vi "Camera_Crop_X_Axis.vi"(9 "Detect Movement":bool, 10 "Camera":T1, 11 "input cluster":T2 {"SystemVersion" items=["Standard", "XL"]; "Overlay_Ring" items=["Session Data", "Extended Setup", "Buffer", "Camera", "Dispenser", "Stats", "Connections"]; "Flush Size" min=1; "Dispense Speed" min=1; "Rectangle 2"."Rotation" format="%.2f"; "Rectangle 2"."Left" scale=0.0..1024.0; "Rectangle 2"."Right" scale=0.0..1024.0; "Rectangle 1"."Rotation" format="%.2f"; "Rectangle 1"."Left" scale=0.0..1024.0; "Rectangle 1"."Right" scale=0.0..1024.0; "Max Framerate" min=1; "Overload threshold" min=1; "Image Save Queue Size" min=1; "Image Process Queue Size" min=1; "Empty start" min=1; "Sample size threshold" min=1; "Framerate" min=1; "Light intensity" scale=0.0..100.0}) -> (1 "Width":i64, 3 "OffsetX":i64)   [LabVIEW 2021]
uses:
  controls/Data.ctl
  <vilib>/userDefined/High Color/IMAQdx.ctl
  <vilib>/vision/Image Controls.llb/IMAQ Image.ctl
  Camera_ID.ctl
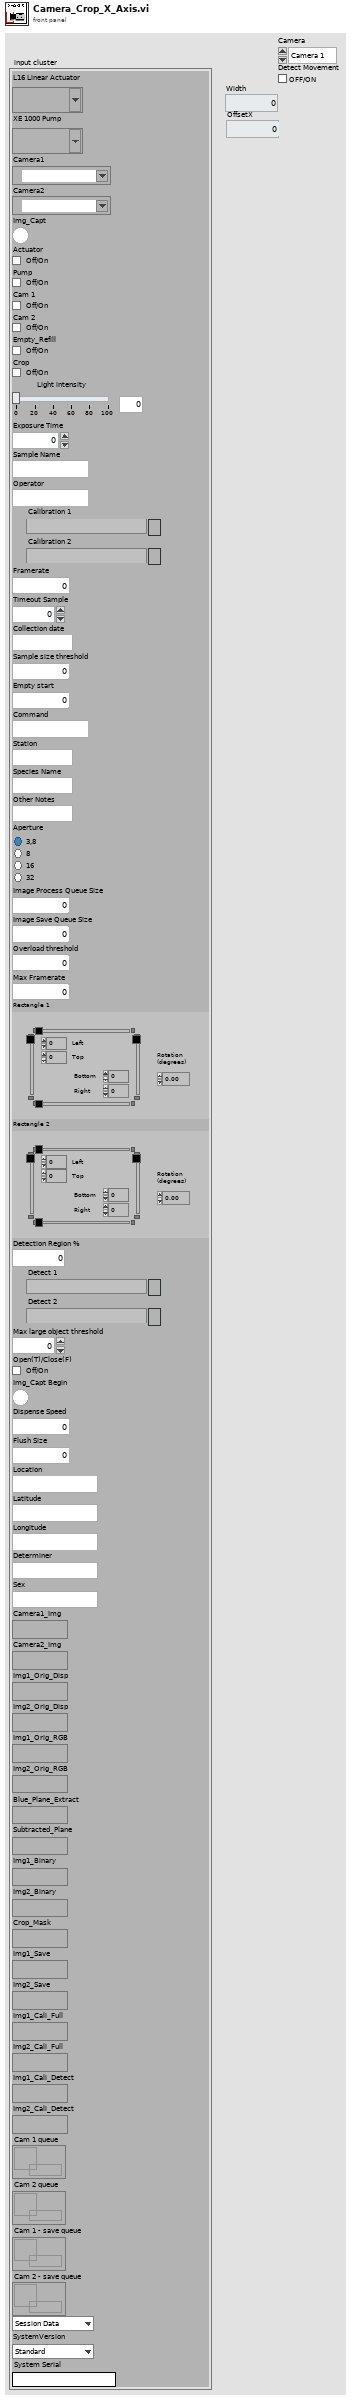
[diagram p1: front panel]
types:
  T1 = typedef "Camera_ID.ctl" = enum16{"Camera 1", "Camera 2"}
  T2 = typedef "Data.ctl" = cluster{"L16 Linear Actuator":refnum<visa-resource-name>, "XE 1000 Pump":refnum<visa-resource-name>, "Camera1":T3, "Camera2":T3, "Img_Capt":bool, "Actuator":bool, "Pump":bool, "Cam 1":bool, "Cam 2":bool, "Empty_Refill":bool, "Crop":bool, "Light intensity":i32, "Exposure Time":dbl, "Sample Name":string, "Operator":string, "Calibration 1":path, "Calibration 2":path, "Framerate":i32, "Timeout Sample":i32, "Collection date":string, "Sample size threshold":i32, "Empty start":u32, "Command":string, "Station":string, "Species Name":string, "Other Notes":string, "Aperture":enum32{"Item 0", "Item 1", "Item 2", "Item 3"}, "Image Process Queue Size":i32, "Image Save Queue Size":i32, "Overload threshold":i32, "Max Framerate":i32, "Rectangle 1":T4, "Rectangle 2":T4, "Detection Region %":dbl, "Detect 1":path, "Detect 2":path, "Max large object threshold":i32, "Open(T)/Close(F)":bool, "Img_Capt Begin":bool, "Dispense Speed":i32, "Flush Size":i32, "Location":string, "Latitude":string, "Longitude":string, "Determiner":string, "Sex":string, "Camera1_Img":T5, "Camera2_Img":T5, "Img1_Orig_Disp":T5, "Img2_Orig_Disp":T5, "Img1_Orig_RGB":T5, "Img2_Orig_RGB":T5, "Blue_Plane_Extract":T5, "Subtracted_Plane":T5, "Img1_Binary":T5, "Img2_Binary":T5, "Crop_Mask":T5, "Img1_Save":T5, "Img2_Save":T5, "Img1_Cali_Full":T5, "Img2_Cali_Full":T5, "Img1_Cali_Detect":T5, "Img2_Cali_Detect":T5, "Cam 1 queue":refnum<queue>, "Cam 2 queue":refnum<queue>, "Cam 1 - save queue":refnum<queue>, "Cam 2 - save queue":refnum<queue>, "Overlay_Ring":u16, "SystemVersion":u16, "System Serial":string}
  T3 = typedef "IMAQdx.ctl" = refnum<k21>
  T4 = typedef "IMAQ Rectangle" = cluster{"Left":i32, "Top":i32, "Right":i32, "Bottom":i32, "Rotation":dbl}
  T5 = typedef "IMAQ Image.ctl" = refnum<image>
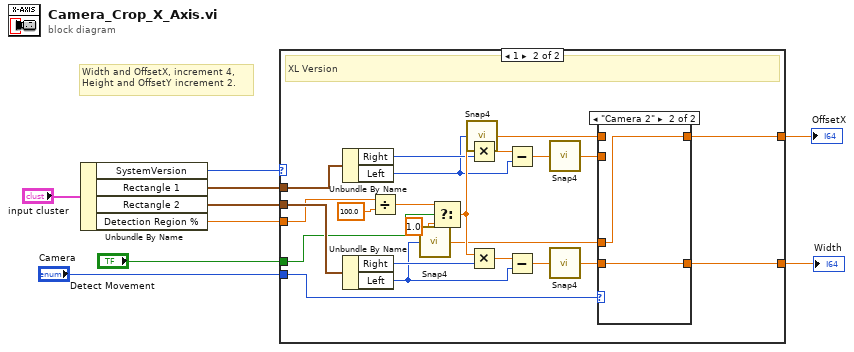
[diagram p0: block diagram]
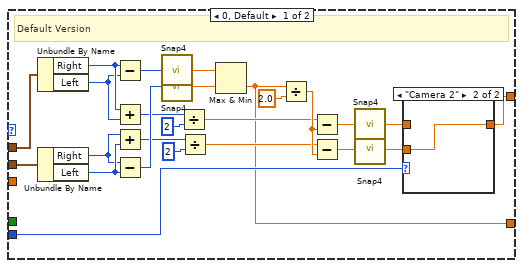
[diagram p2: hidden frame]
diagram:
  # "Width and OffsetX, increment 4,\nHeight and OffsetY increment 2."
  n1 = Unbundle By Name("input cluster") -> ("SystemVersion"=w5:u16, "Rectangle 1"=w7:T4, "Rectangle 2"=w8:T4, "Detection Region %"=w4:dbl)
  n2 = case shown="1" w5 {
    tunnel: w8 -> [w26 w44]
    tunnel: w7 -> [w20 w45]
    tunnel: "Camera" -> [w18 w41]
    tunnel: [w14 w39] -> w1
    tunnel: [w15 w40] -> w2
    tunnel: w4 -> [_ w43]
    tunnel: "Detect Movement" -> [_ w42]
    frame 0, Default {
      # "Default Version"
      n3 = Unbundle By Name(w20) -> ("Right"=w11:i32, "Left"=w10:i32)
      n4 = Unbundle By Name(w26) -> ("Right"=w12:i32, "Left"=w13:i32)
      n5 = Subtract(x=w11, y=w10) -> (x-y=w29:i32)
      n6 = Add(x=w11, y=w10) -> (x+y=w21:i32)
      n7 = Add(x=w12, y=w13) -> (x+y=w24:i32)
      n8 = Subtract(x=w12, y=w13) -> (x-y=w32:i32)
      n9 = call "Snap4.vi"("x"=w29) -> ("x out"=w30:dbl)
      n10 = call "Snap4.vi"("x"=w32) -> ("x out"=w33:dbl)
      n11 = Divide(x=w21, y=2) -> (x/y=w23:dbl)
      n12 = Divide(x=w24, y=2) -> (x/y=w27:dbl)
      n13 = Max & Min(x=w30, y=w33) -> (min(x,y)=w14:dbl)  [unwired: 1 out]
      n14 = Divide(x=w14, y=2.0) -> (x/y=w28:dbl)
      n15 = Subtract(x=w23, y=w28) -> (x-y=w31:dbl)
      n16 = Subtract(x=w27, y=w28) -> (x-y=w34:dbl)
      n17 = call "Snap4.vi"("x"=w31) -> ("x out"=w17:dbl)
      n18 = call "Snap4.vi"("x"=w34) -> ("x out"=w16:dbl)
      n19 = case shown="\"Camera 2\"" w18 {
        tunnel: w17 -> [w35 _]
        tunnel: [w35 w36] -> w15
        tunnel: w16 -> [_ w36]
        frame "Camera 1", Default {
        }
        frame "Camera 2" {
        }
      }
    }
    frame 1 {
      # "XL Version"
      n20 = Unbundle By Name(w45) -> ("Right"=w50:i32, "Left"=w38:i32)
      n21 = Unbundle By Name(w44) -> ("Right"=w52:i32, "Left"=w37:i32)
      n22 = Divide(x=w43, y=100.0 ("x")) -> (x/y=w56:dbl)
      n23 = call "Snap4.vi"("x"=w37) -> ("x out"=w49:dbl)
      n24 = Select(t=w56, s=w42, f=1.0 ("t")) -> (s? t:f=w54:dbl)
      n25 = call "Snap4.vi"("x"=w38) -> ("x out"=w47:dbl)
      n26 = Multiply(x=w54, y=w50) -> (x*y=w51:dbl)
      n27 = Multiply(x=w54, y=w52) -> (x*y=w53:dbl)
      n28 = Subtract(x=w51, y=w38) -> (x-y=w58:dbl)
      n29 = Subtract(x=w53, y=w37) -> (x-y=w59:dbl)
      n30 = call "Snap4.vi"("x"=w58) -> ("x out"=w46:dbl)
      n31 = call "Snap4.vi"("x"=w59) -> ("x out"=w48:dbl)
      n32 = case shown="\"Camera 2\"" w41 {
        tunnel: w49 -> [_ w63]
        tunnel: [w61 w63] -> w40
        tunnel: w46 -> [w60 _]
        tunnel: [w60 w62] -> w39
        tunnel: w47 -> [w61 _]
        tunnel: w48 -> [_ w62]
        frame "Camera 1", Default {
        }
        frame "Camera 2" {
        }
      }
    }
  }
  "Width" <- w1
  "OffsetX" <- w2
